vi "Layer.vi"(8 "Index":i32, 9 "Thickness":dbl, 10 "Contours":T1[](array[typedef]), 11 "DocIn":refnum<k20>) -> (2 "Layer":refnum<k20>, 3 "DocOut":refnum<k20>)   [LabVIEW 2014]
uses:
  TypeDefs/Poly2DwSlope.ctl
  TypeDefs/Point2DwSlope.ctl
  <resource>/objmgr/DOMUserDefRef.rc
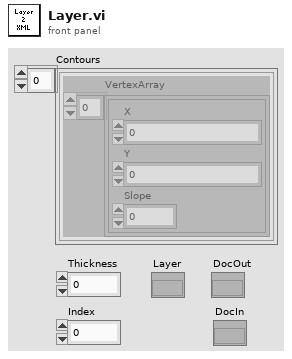
[diagram p1: front panel]
types:
  T1 = typedef "Poly2DwSlope.ctl" = cluster{"VertexArray":T2[]}
  T2 = typedef "Point2DwSlope.ctl" = cluster{"X":sgl, "Y":sgl, "Slope":dbl}
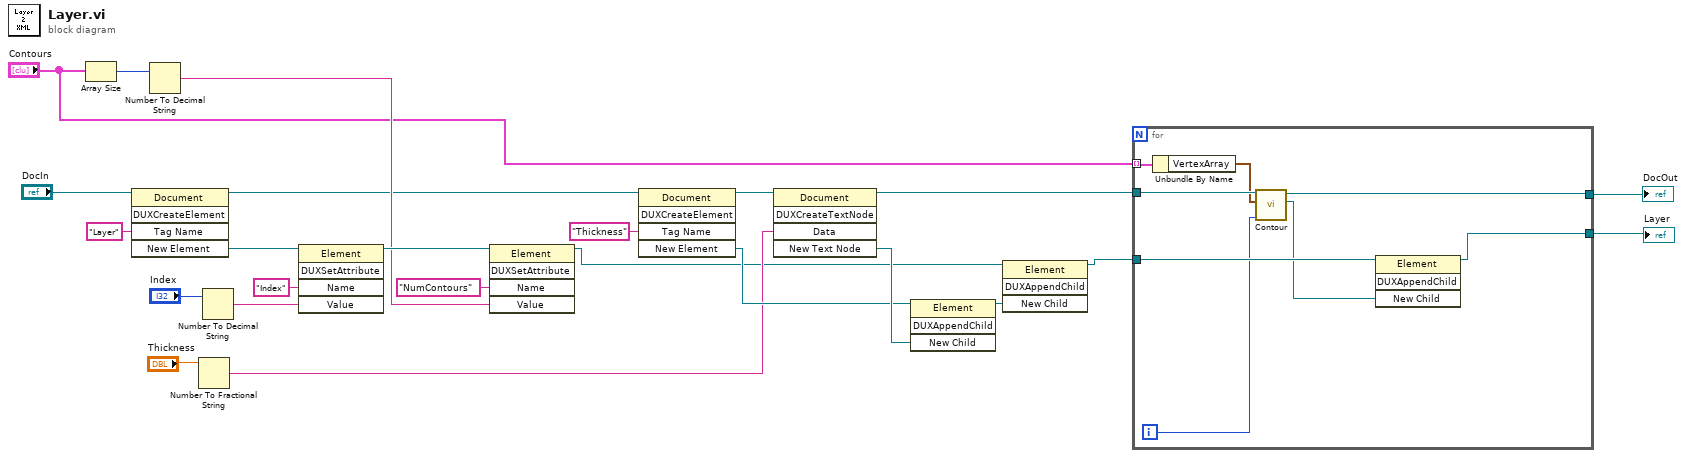
[diagram p0: block diagram]
diagram:
  n1 = Array Size(array="Contours") -> (size(s)=w17:i32)
  n2 = invoke class="Document" method="DUXCreateElement"(reference="DocIn", "Tag Name"="Layer") -> (reference out=w9:refnum<k20>, "New Element"=w20:refnum<k20>)  [unwired: 3 in, 3 out]
  n3 = Number To Decimal String(number=w17) -> (decimal integer string=w16:string)  [unwired: 1 in]
  n4 = Number To Fractional String(number="Thickness") -> (F-format string=w6:string)  [unwired: 3 in]
  n5 = Number To Decimal String(number="Index") -> (decimal integer string=w22:string)  [unwired: 1 in]
  n6 = invoke class="Element" method="DUXSetAttribute"(reference=w20, "Name"="Index", "Value"=w22) -> (reference out=w19:refnum<k20>)  [unwired: 2 in, 4 out]
  n7 = invoke class="Element" method="DUXSetAttribute"(reference=w19, "Name"="NumContours", "Value"=w16) -> (reference out=w5:refnum<k20>)  [unwired: 2 in, 4 out]
  n8 = invoke class="Document" method="DUXCreateElement"(reference=w9, "Tag Name"="Thickness") -> (reference out=w13:refnum<k20>, "New Element"=w11:refnum<k20>)  [unwired: 3 in, 3 out]
  n9 = invoke class="Document" method="DUXCreateTextNode"(reference=w13, "Data"=w6) -> (reference out=w8:refnum<k20>, "New Text Node"=w12:refnum<k20>)  [unwired: 3 in, 3 out]
  n10 = invoke class="Element" method="DUXAppendChild"(reference=w11, "New Child"=w12) -> (reference out=w10:refnum<k20>)  [unwired: 2 in, 3 out]
  n11 = invoke class="Element" method="DUXAppendChild"(reference=w5, "New Child"=w10) -> (reference out=w4:refnum<k20>)  [unwired: 2 in, 3 out]
  n12 = for {
    tunnel: w8 -> [w32]
    tunnel: "Contours" -> [w31] mode=indexing
    tunnel: w4 -> [w29]
    tunnel: [w26] -> w2
    tunnel: [w25] -> w3
    i -> [w27]
    n13 = Unbundle By Name(w31) -> ("VertexArray"=w30:T2[])
    n14 = call "Contour.vi"("Index"=w27, "VertexArray"=w30, "DocIn"=w32) -> ("Contour"=w28:refnum<k20>, "DocOut"=w26:refnum<k20>)  [unwired: 7 in]
    n15 = invoke class="Element" method="DUXAppendChild"(reference=w29, "New Child"=w28) -> (reference out=w25:refnum<k20>)  [unwired: 2 in, 3 out]
  }
  "Layer" <- w3
  "DocOut" <- w2
